vi "WT-Sensor_Data-Viewer.vi"() -> ()   [LabVIEW 2017]
uses:
  <vilib>/Utility/file.llb/Write Delimited Spreadsheet (DBL).vi
panel:
  in  "Sampling Frequency (Hz)":sgl=5000.0
  in  "Record_Data":bool caption="Record Data:"
  out "HeartBeat":bool
  out "Path":path caption="File Path:"
  out "ElapsedTime":string caption="Elapsed Time:"
  out "StratTime":string caption="Strat Time:"
  out "MWTV":dbl(graph) caption="Main Wind Tunnel Velocity"
  out "LATD":dbl(graph) caption="Lab Atmospheric Density"
  out "LATT":dbl(graph) caption="Lab Atmospheric Temperature"
  out "LATP":dbl(graph) caption="Lab Atmospheric Pressure"
  out "MWTP":dbl(graph) caption="Main Wind Tunnel Pressure"
  in  "Stop":bool caption="Log Data:"
  # "Wind Tunnel Sensor Data Viewer"
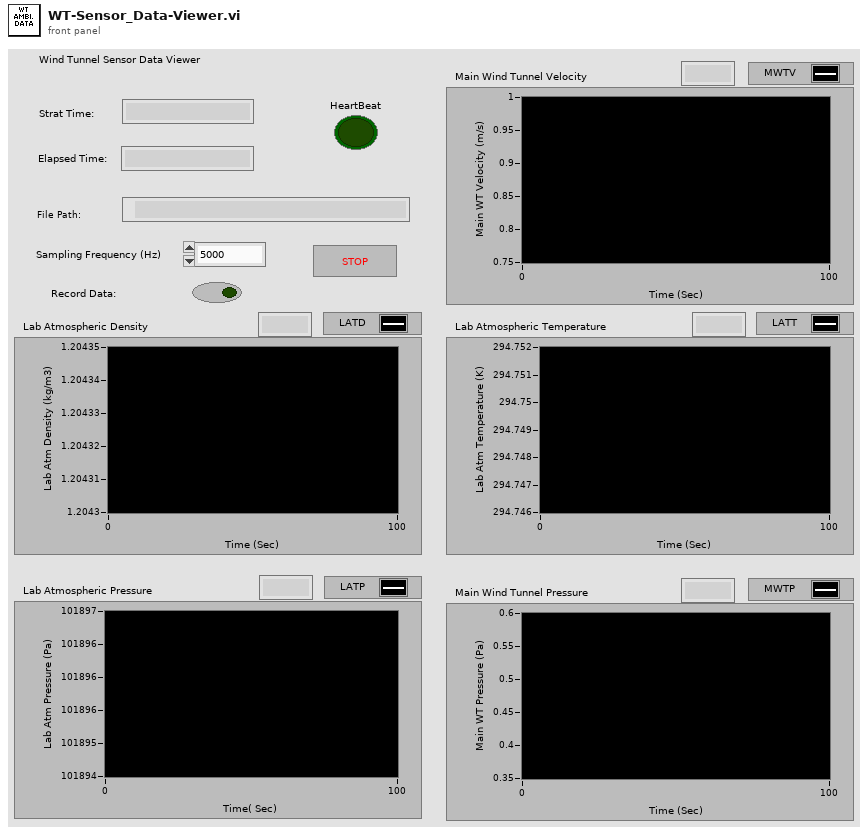
[diagram p1: front panel]
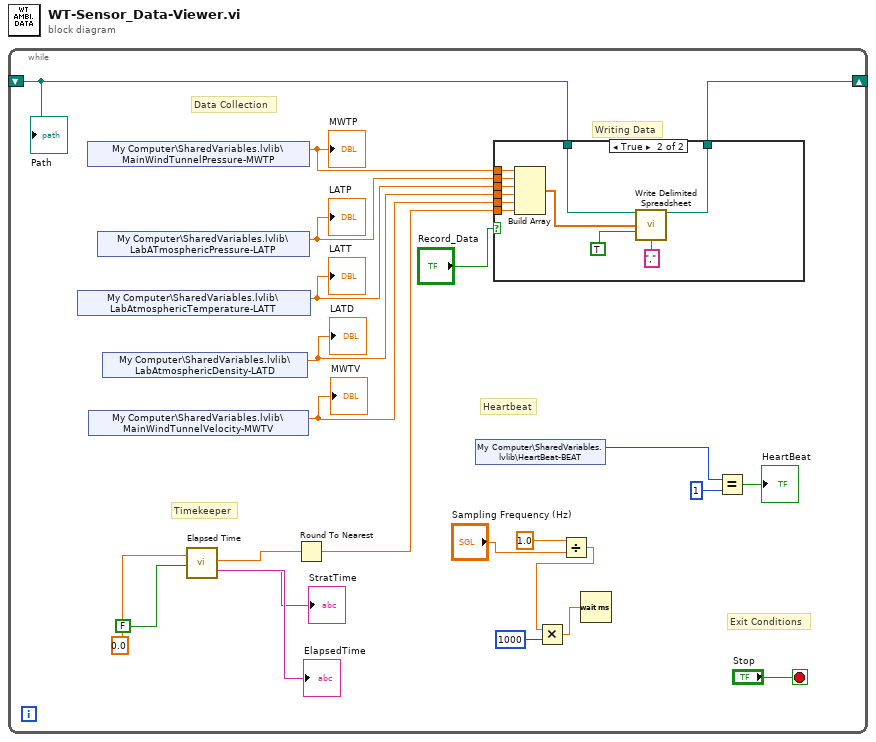
[diagram p0: block diagram]
diagram:
  n1 = while {
    shift-right: [w18] -> _
    shift-left: _ -> [w7]
    stop <- "Stop" stop-if-true
    # "Heartbeat"
    # "Exit Conditions"
    # "Writing Data"
    # "Data Collection"
    # "Timekeeper"
    n2 = shared-variable "My Computer\\SharedVariables.lvlib\\LabAtmosphericTemperature-LATT"() -> (w21:dbl)  [unwired: 1 in, 1 out]
    "LATT" <- w21
    n3 = shared-variable "My Computer\\SharedVariables.lvlib\\MainWindTunnelPressure-MWTP"() -> (w20:dbl)  [unwired: 1 in, 1 out]
    "MWTP" <- w20
    n4 = shared-variable "My Computer\\SharedVariables.lvlib\\MainWindTunnelVelocity-MWTV"() -> (w16:dbl)  [unwired: 1 in, 1 out]
    "MWTV" <- w16
    n5 = shared-variable "My Computer\\SharedVariables.lvlib\\LabATmosphericPressure-LATP"() -> (w19:dbl)  [unwired: 1 in, 1 out]
    "LATP" <- w19
    n6 = shared-variable "My Computer\\SharedVariables.lvlib\\LabAtmosphericDensity-LATD"() -> (w17:dbl)  [unwired: 1 in, 1 out]
    "LATD" <- w17
    n7 = call "Elapsed Time"("Auto Reset"=FALSE, "Set Start Time (s)"=0.0) -> ("Start Time Text"=→"StratTime":string, "Elapsed Time (s)"=w22:dbl, "Elapsed Time Text"=→"ElapsedTime":string)  [unwired: 10 in, 5 out]
    n8 = Round To Nearest(number=w22) -> (nearest integer value=w23:dbl)
    n9 = shared-variable "My Computer\\SharedVariables.lvlib\\HeartBeat-BEAT"() -> (w11:i8)  [unwired: 1 in, 1 out]
    n10 = case shown="True" "Record_Data" {
      tunnel: w23 -> [_ w32]
      tunnel: w7 -> [w24 w31]
      tunnel: w21 -> [_ w30]
      tunnel: w20 -> [_ w29]
      tunnel: w19 -> [_ w28]
      tunnel: [w24 w27] -> w18
      tunnel: w17 -> [_ w26]
      tunnel: w16 -> [_ w25]
      frame False {
      }
      frame True {
        n11 = Build Array(w29, w28, w30, w26, w25, w32) -> (w33:dbl[])
        n12 = call-poly <vilib>:"Write Delimited Spreadsheet.vi"("file path (dialog if empty)"=w31, "1D data"=w33, "append to file? (new file:F)"=TRUE, "delimiter (\\t)"="," ("delimiter (\\t)")) -> ("new file path (Not A Path if cancelled)"=w27:path)  [unwired: 10 in, 1 out]
      }
    }
    n13 = Divide(x=sgl 1.0, y="Sampling Frequency (Hz)") -> (x/y=w1:sgl)
    n14 = Multiply(x=w1, y=u32 1000) -> (x*y=w4:sgl)
    n15 = Wait (ms)(milliseconds to wait=w4) -> ()  [unwired: 1 out]
    n16 = Equal?(x=w11, y=i8 1 ("x")) -> (x = y?=→"HeartBeat":bool)
    "Path" <- w7
  }
